vi "FRCts20_Backend_API_RequestRoot.vi"(8 "error in (no error)":errorcluster, 10 "Message":T1="GetRequestRoot", 11 "Request In":T2) -> (0 "error out":errorcluster, 2 "Status":string, 3 "Request Out":T2)   [LabVIEW 2014, in "FRCts20_Backend_API.lvlib"]
doc: "This API call retrieves information for all requests or creates a new request"
uses:
  FRCts20_Backend_API.lvlib
  FRCts20_Backend_API_RequestRoot.ctl
  FRCts20_Backend_API_Status.ctl
  FRCts20_Backend_API_Command_RequestRoot.ctl
  FRCts20_Backend_FGVOperation.ctl
  FRCts20_Backend_Engine.lvlib
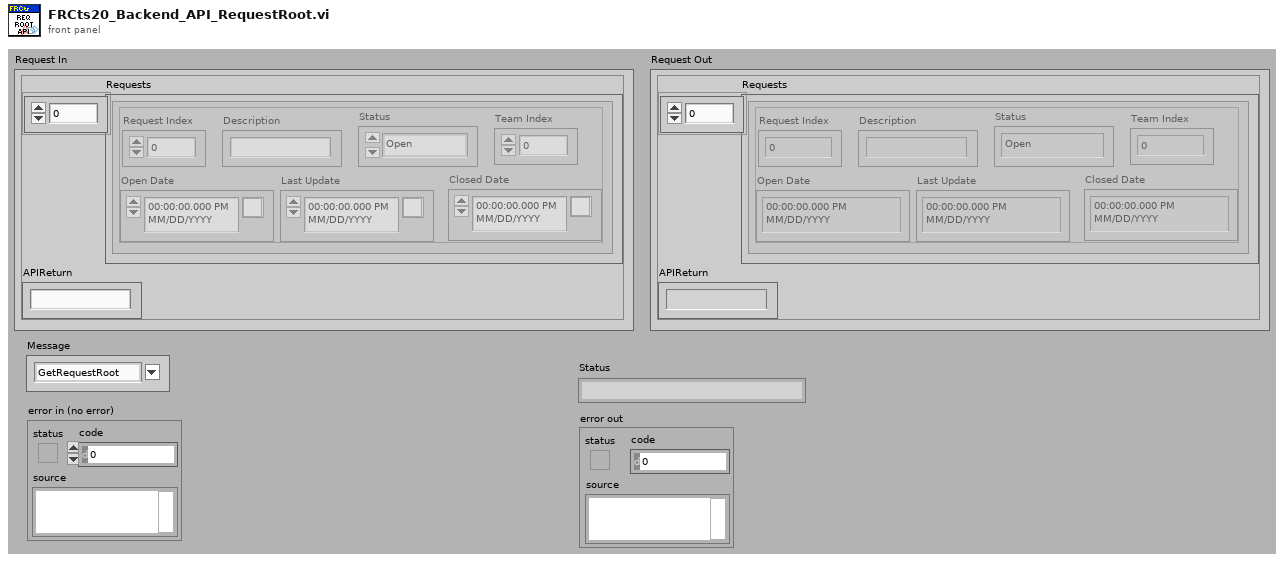
[diagram p1: front panel]
types:
  T1 = typedef "FRCts20_Backend_API.lvlib/FRCts20_Backend_API_Command_RequestRoot.ctl" = string
  T2 = typedef "FRCts20_Backend_API.lvlib/FRCts20_Backend_API_RequestRoot.ctl" = cluster{"Requests":cluster{"Request Index":u32, "Description":string, "Status":T3, "Open Date":timestamp, "Last Update":timestamp, "Closed Date":timestamp, "Team Index":u32}[], "APIReturn":string}
  T3 = typedef "FRCts20_Backend_API.lvlib/FRCts20_Backend_API_Status.ctl" = enum16{"Open", "In Work", "Closed"}
  T4 = typedef "FRCts20_Backend_Engine.lvlib/FRCts20_Backend_FGVOperation.ctl" = enum16{"Initialize", "EnqueueMessage", "EnqueueDataReturn", "FlushMessage", "FlushDataReturn"}
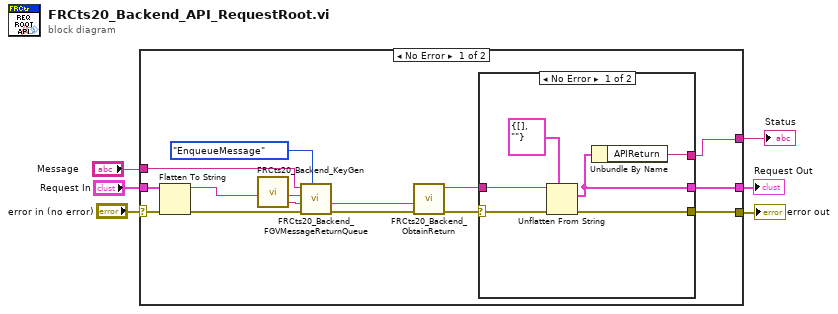
[diagram p0: block diagram]
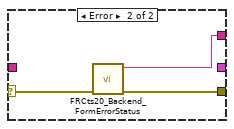
[diagram p2: hidden frame]
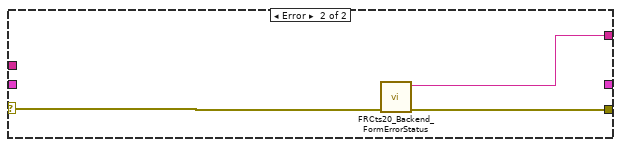
[diagram p3: hidden frame]
diagram:
  n1 = case shown="No Error" "error in (no error)" {
    selector: "error in (no error)" -> [w19 w32]
    tunnel: [w9 w31] -> w5
    tunnel: [w11 w30] -> w4
    tunnel: "Message" -> [w15 _]
    tunnel: "Request In" -> [w14 _]
    tunnel: [w10 _] -> w1
    frame No Error {
      n2 = Flatten To String(anything=w14, error in (no error)=w19) -> (data string=w20:string, error out=w18:errorcluster)  [unwired: 2 in, 1 out]
      n3 = call "FRCts20_Backend_KeyGen.vi"() -> ("Keygen"=w17:string)  [unwired: 27 in]
      n4 = call "FRCts20_Backend_FGVMessageReturnQueue.vi"("Operation"=FRCts20_Backend_FGVOperation."EnqueueMessage", "error in (no error)"=w18, "Key"=w17, "Message Value"=w20, "Message Name"=w15) -> ("error out"=w8:errorcluster, "Key (Duplicate)"=w7:string)  [unwired: 5 in]
      n5 = call "FRCts20_Backend_ObtainReturn.vi"("error in (no error)"=w8, "Key"=w7) -> ("error out"=w12:errorcluster, "Message Value"=w13:string)  [unwired: 8 in]
      n6 = case shown="No Error" w12 {
        selector: w12 -> [w25 w29]
        tunnel: [w26 w28] -> w9
        tunnel: [w24 _] -> w10
        tunnel: [w23 w27] -> w11
        tunnel: w13 -> [w22 _]
        frame No Error {
          n7 = Unflatten From String(type=T2 {"Requests"=[], "APIReturn"=""} ("Request"), binary string=w22, error in (no error)=w25) -> (value=w24:T2, error out=w26:errorcluster)  [unwired: 2 in, 1 out]
          n8 = Unbundle By Name(w24) -> ("APIReturn"=w23:string)
        }
        frame Error {
          n9 = call "FRCts20_Backend_FormErrorStatus.vi"("error in (no error)"=w29) -> ("error out"=w28:errorcluster, "String"=w27:string)  [unwired: 9 in]
        }
      }
    }
    frame Error {
      n10 = call "FRCts20_Backend_FormErrorStatus.vi"("error in (no error)"=w32) -> ("error out"=w31:errorcluster, "String"=w30:string)  [unwired: 9 in]
    }
  }
  "error out" <- w5
  "Status" <- w4
  "Request Out" <- w1
